vi "Z_CONT (M).vi"(8 "error in (no error)":errorcluster, 9 "element":T1 {"Avoid zero threshold (V)" format="%#_13g"}, 10 "ScanQ in":refnum<queue>, 11 "SweepQ In":refnum<queue>) -> (0 "error out":errorcluster, 1 "SweepQ Out":refnum<queue>, 2 "Z-Controller on/off status":bool, 3 "Queue out":refnum<queue>)   [LabVIEW 2025]
uses:
  STM-Auto-Project/QMH CTLS/Scan_Params (QMH).ctl
  <userlib>/Nanonis Prog Interface V5e/Nanonis Prog Interface.lvlib
  LabVIEW VI's/Instrument VI's/Instrument Controls/Magnet Array.ctl
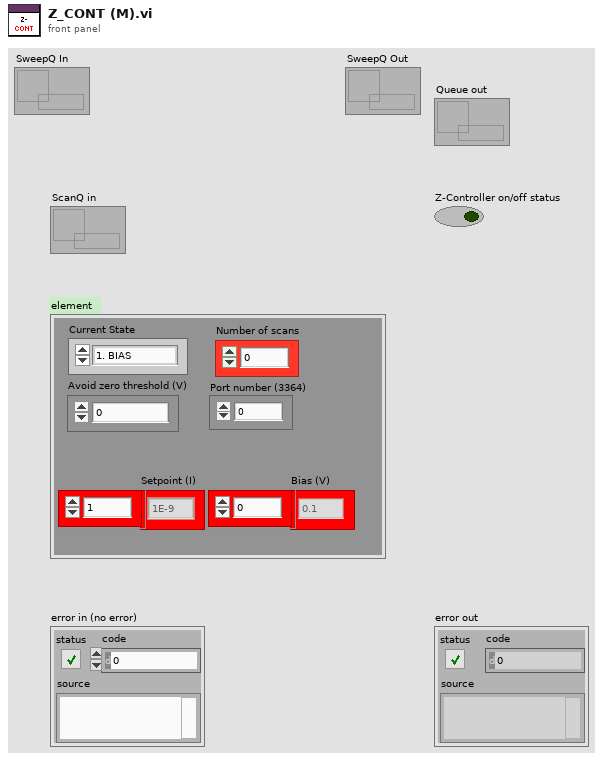
[diagram p1: front panel]
types:
  T1 = typedef "Scan_Params (QMH).ctl" = cluster{"Setpoint (I)":dbl[], "Bias (V)":dbl[], "Number of scans":u8, "Port number (3364)":u32, "Avoid zero threshold (V)":dbl, "Current State":enum16{"1. BIAS", "2. INIT_SCAN", "3. SCAN_IDLE", "4. INTER_SCAN", "5. NEW_COORDS_&_FRAME", "6. FINAL_SCAN", "7. POLL BIAS ", "8. Z-CONT.", "9. STOP"}}
  T2 = enum16{"1. BIAS", "2. INIT_SCAN", "3. SCAN_IDLE", "4. INTER_SCAN", "5. NEW_COORDS_&_FRAME", "6. FINAL_SCAN", "7. POLL BIAS ", "8. Z-CONT.", "9. STOP"}
  T3 = enum16{"SET FIELD", "SWEEP IDLE", "NEXT FIELD", "SWEEP DONE"}
  T4 = typedef "Magnet Array.ctl" = cluster{"Sweep States":enum16{"SET FIELD", "SWEEP IDLE", "NEXT FIELD", "SWEEP DONE"}, "VISA Connection":refnum<visa-resource-name>, "Fields(T)":dbl[]}
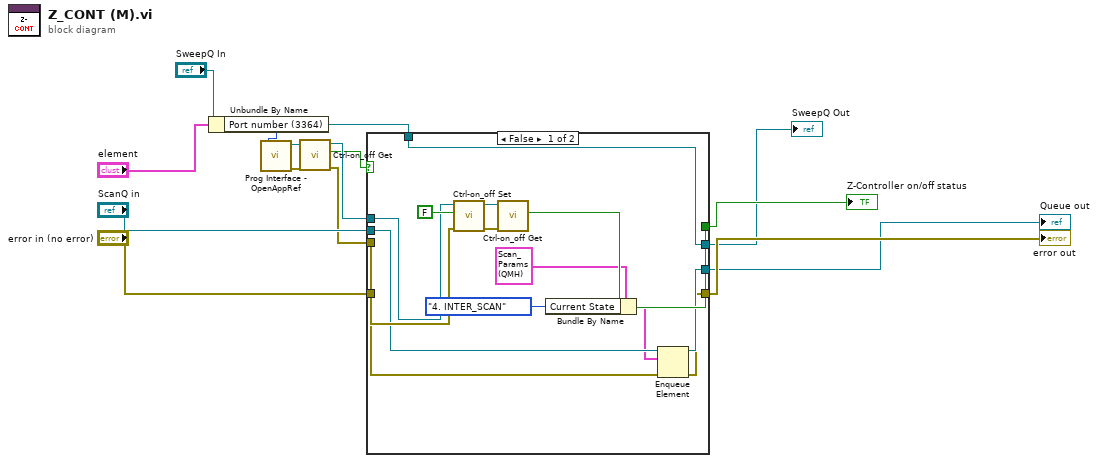
[diagram p0: block diagram]
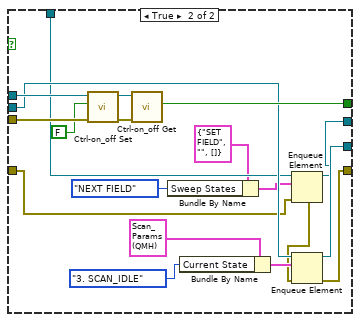
[diagram p2: hidden frame]
diagram:
  n1 = Unbundle By Name("element") -> ("Port number (3364)"=w14:u32)
  n2 = call <userlib>:"Prog Interface - OpenAppRef.vi"("Port number (3364)"=w14) -> ("Error out"=w11:errorcluster, "Application reference"=w12:refnum<vi>)  [unwired: 5 in]
  n3 = call <userlib>:"Ctrl-on_off Get.vi"("error in (no error)"=w11, "Application ref in"=w12) -> ("error out"=w5:errorcluster, "Z-Controller on/off status"=w3:bool, "Application ref out"=w4:refnum<vi>)  [unwired: 7 in]
  n4 = case shown="False" w3 {
    tunnel: w4 -> [w25 w47]
    tunnel: w5 -> [w24 w46]
    tunnel: [w23 w42] -> w6
    tunnel: "ScanQ in" -> [w22 w41]
    tunnel: [w18 w37] -> w8
    tunnel: [w17 w36] -> w9
    tunnel: "error in (no error)" -> [w16 w34]
    tunnel: [w15 w32] -> w2
    tunnel: "SweepQ In" -> [w15 w31]
    frame False {
      n5 = call <userlib>:"Ctrl-on_off Set.vi"("error in (no error)"=w24, "Z Controller ON/OFF"=FALSE, "Application ref in"=w25) -> ("error out"=w27:errorcluster, "Application ref out"=w26:refnum<vi>)  [unwired: 7 in]
      n6 = call <userlib>:"Ctrl-on_off Get.vi"("error in (no error)"=w27, "Application ref in"=w26) -> ("Z-Controller on/off status"=w23:bool)  [unwired: 7 in, 2 out]
      n7 = Bundle By Name(cluster=T1 {"Setpoint (I)"=[], "Bias (V)"=[], "Number of scans"=1, "Port number (3364)"=3364, "Avoid zero threshold (V)"=0.004999999888241291, "Current State"=enum."1. BIAS"} ("element"), "Current State"=T2."4. INTER_SCAN") -> (w20:T1)
      n8 = Enqueue Element(queue=w22, element=w20, error in (no error)=w16) -> (queue out=w18:refnum<queue>, error out=w17:errorcluster)  [unwired: 1 in, 1 out]
    }
    frame True {
      n9 = call <userlib>:"Ctrl-on_off Set.vi"("error in (no error)"=w46, "Z Controller ON/OFF"=FALSE, "Application ref in"=w47) -> ("error out"=w44:errorcluster, "Application ref out"=w43:refnum<vi>)  [unwired: 7 in]
      n10 = call <userlib>:"Ctrl-on_off Get.vi"("error in (no error)"=w44, "Application ref in"=w43) -> ("Z-Controller on/off status"=w42:bool)  [unwired: 7 in, 2 out]
      n11 = Bundle By Name(cluster=T4 {"Sweep States"=enum."SET FIELD", "VISA Connection"="", "Fields(T)"=[]} ("element"), "Sweep States"=T3."NEXT FIELD") -> (w35:T4)
      n12 = Bundle By Name(cluster=T1 {"Setpoint (I)"=[], "Bias (V)"=[], "Number of scans"=1, "Port number (3364)"=3364, "Avoid zero threshold (V)"=0.004999999888241291, "Current State"=enum."1. BIAS"} ("element"), "Current State"=T2."3. SCAN_IDLE") -> (w39:T1)
      n13 = Enqueue Element(queue=w31, element=w35, error in (no error)=w34) -> (queue out=w32:refnum<queue>, error out=w33:errorcluster)  [unwired: 1 in, 1 out]
      n14 = Enqueue Element(queue=w41, element=w39, error in (no error)=w33) -> (queue out=w37:refnum<queue>, error out=w36:errorcluster)  [unwired: 1 in, 1 out]
    }
  }
  "error out" <- w9
  "Queue out" <- w8
  "Z-Controller on/off status" <- w6
  "SweepQ Out" <- w2
